vi "UpdateFeatureStudio.vi"(0 "Device In":T2, 5 "did":string, 7 "wid":string, 9 "eid":string, 11 "error in":errorcluster, 12 "FeatureScript":string) -> (4 "Device Out":T2, 6 "Comm":T1, 15 "error out":errorcluster)   [LabVIEW 2019]
uses:
  <userlib>/IoT Devices/_subVIs/HTTPComm.ctl
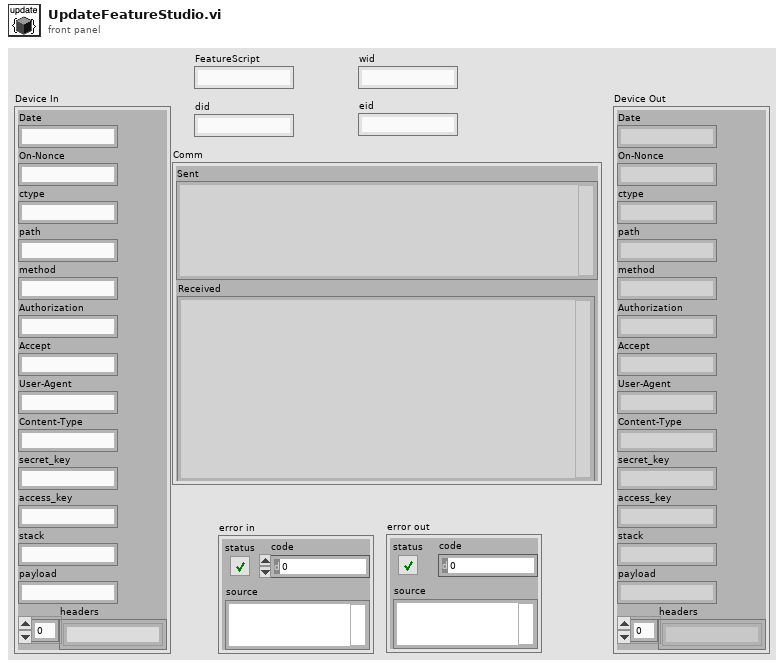
[diagram p1: front panel]
types:
  T1 = typedef "HTTPComm.ctl" = cluster{"url":string, "sent headers":string, "sent body":string, "headers":string, "body":string, "Sent":string, "Received":string}
  T2 = cluster{"Date":string, "On-Nonce":string, "ctype":string, "path":string, "method":string, "Authorization":string, "Accept":string, "User-Agent":string, "Content-Type":string, "secret_key":string, "access_key":string, "stack":string, "payload":string, "headers":string[]}
  T3 = cluster{"contents":string, "serializationVersion":string, "sourceMicroversion":string, "rejectMicroversionSkew":bool}
  T4 = cluster{"contents":string, "serializationVersion":string, "sourceMicroversion":string, "rejectMicroversionSkew":bool, "microversionSkew":bool, "libraryVersion":i32}
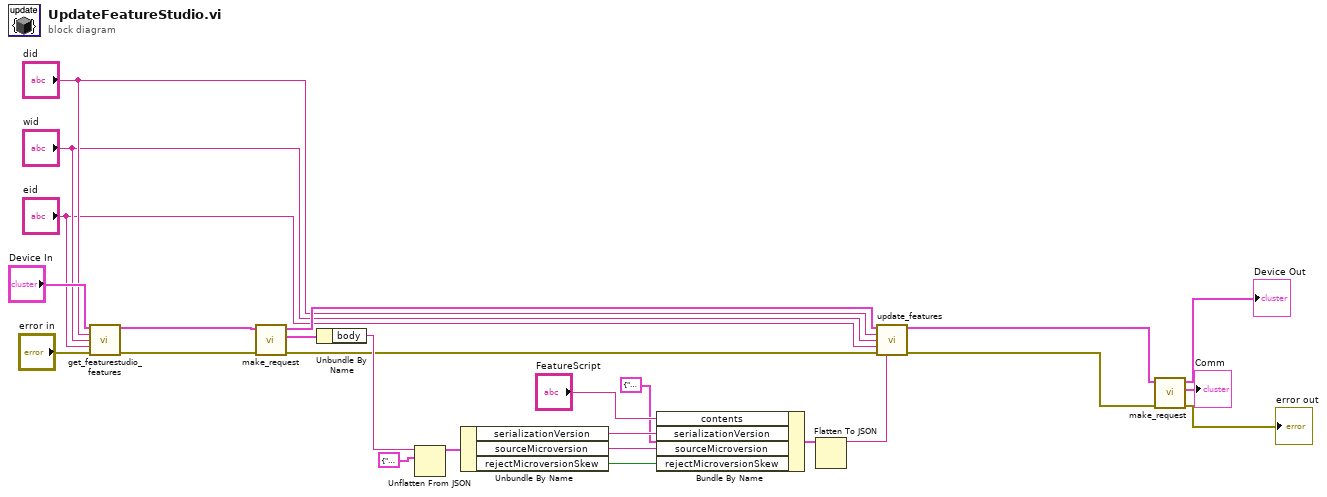
[diagram p0: block diagram]
diagram:
  n1 = call <userlib>:"get_featurestudio_features.vi"("Device In"="Device In", "did"="did", "wid"="wid", "eid"="eid", "error in"="error in") -> ("Device Oout"=w16:T2, "error out"=w15:errorcluster)  [unwired: 9 in]
  n2 = call "make_request.vi"("Error in"=w15, "Device In"=w16) -> ("error out"=w10:errorcluster, "Comm"=w14:T1, "Device Out"=w9:T2)  [unwired: 7 in]
  n3 = Unbundle By Name(w14) -> ("body"=w13:string)
  n4 = Unflatten From JSON(JSON string=w13, type and defaults=T4 {"contents"="", "serializationVersion"="", "sourceMicroversion"="", "rejectMicroversionSkew"=TRUE, "microversionSkew"=TRUE, "libraryVersion"=0}) -> (value=w21:T4)  [unwired: 5 in, 1 out]
  n5 = Unbundle By Name(w21) -> ("serializationVersion"=w22:string, "sourceMicroversion"=w23:string, "rejectMicroversionSkew"=w24:bool)
  n6 = Bundle By Name(cluster=T3 {"contents"="", "serializationVersion"="", "sourceMicroversion"="", "rejectMicroversionSkew"=TRUE}, "contents"="FeatureScript", "serializationVersion"=w22, "sourceMicroversion"=w23, "rejectMicroversionSkew"=w24) -> (w19:T3)
  n7 = Flatten To JSON(anything=w19) -> (JSON string=w11:string)  [unwired: 2 in, 1 out]
  n8 = call <userlib>:"update_features.vi"("Device In"=w9, "did"="did", "wid"="wid", "eid"="eid", "error in"=w10, "payload"=w11) -> ("Device Out"=w3:T2, "error out"=w4:errorcluster)  [unwired: 8 in]
  n9 = call "make_request.vi"("Error in"=w4, "Device In"=w3) -> ("error out"=→"error out":errorcluster, "Comm"=→"Comm":T1, "Device Out"=→"Device Out":T2)  [unwired: 7 in]
